vi "Teleop.vi"(10 "Match Info":T1={"Autonomous Elapsed Seconds"=0.0, "TeleOp Elapsed Seconds"=0.0, "Disabled Elapsed Seconds"=0.0, "Visited Autonomous"=FALSE, "Visited TeleOp"=FALSE, "Visited Disabled"=FALSE, "Autonomous Settings"={"Autonomous Style"=enum."Independent", "VI Refnum"=refnum}}, 11 "Call Context":T2) -> ()   [LabVIEW 2019]
doc: "This VI is called for each TeleOp packet received from the DS where the robot is not disabled. It is often used to read from the joysticks and update I/O or to update setpoints for timed control loops. It should complete and return within 20 milliseconds or it may miss DS packets."
uses:
  <vilib>/Rock Robotics/WPI/DriverStation/WPI_DriverStationDerivedRobotMode.ctl
  <vilib>/Rock Robotics/WPI/DriverStation/WPI_DriverStationMatch Info.ctl
  <vilib>/Rock Robotics/WPI/Utilities/WPI_GetSetVariantRefNum.vi
  <vilib>/Rock Robotics/Network Tables/NT Write String.vi
  <vilib>/Rock Robotics/Network Tables/NT Write Number.vi
  <vilib>/Rock Robotics/Network Tables/NT Write Numeric Array.vi
  <vilib>/Rock Robotics/Network Tables/NT Read Boolean.vi
  Robot Global Data.vi
  <vilib>/Rock Robotics/Network Tables/NT Read Number.vi
  <vilib>/Rock Robotics/Network Tables/NT Write Boolean Array.vi
panel:
  in  "Yellow":cluster{"R":dbl, "G":dbl, "B":dbl}
  in  "Blue":cluster{"R":dbl, "G":dbl, "B":dbl}
  in  "Green":cluster{"R":dbl, "G":dbl, "B":dbl}
  in  "Red":cluster{"R":dbl, "G":dbl, "B":dbl}
  in  "None":cluster{"R":dbl, "G":dbl, "B":dbl}
  in  "None":cluster{"R":dbl, "G":dbl, "B":dbl}
  out "Sample Slider 0":dbl(slide) scale=0.0..5.0
  out "Sample Boolean 1":bool
  out "Sample Boolean 0":bool
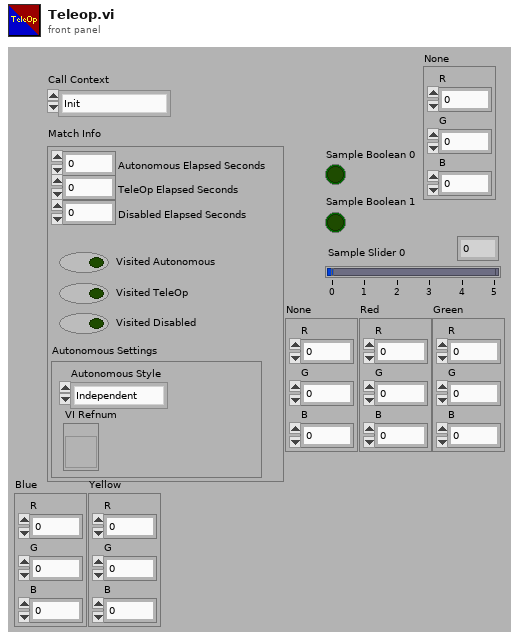
[diagram p1: front panel]
types:
  T1 = typedef "WPI_DriverStationMatch Info.ctl" = cluster{"Autonomous Elapsed Seconds":dbl, "TeleOp Elapsed Seconds":dbl, "Disabled Elapsed Seconds":dbl, "Visited Autonomous":bool, "Visited TeleOp":bool, "Visited Disabled":bool, "Autonomous Settings":cluster{"Autonomous Style":enum16{"Iterative", "Independent"}, "VI Refnum":refnum<vi>}}
  T2 = typedef "WPI_DriverStationDerivedRobotMode.ctl" = enum16{"Init", "Execute", "Stop"}
  T3 = typedef "WPI_RobotDriveDevRef.ctl" = cluster{"DevStatus":errorcluster, "Motors[]":T4[], "Square Inputs":bool, "Max Output":dbl}
  T4 = typedef "WPI_MotorControlDeviceRef.ctl" = cluster{"DeviceStatus":errorcluster, "Type":T5, "PWM":cluster{"PWM Channel":T6, "DeadBand":T7}, "CAN":cluster{"Device Number":u8, "SetOutput VI Ref":variant, "GetOutput VI Ref":variant, "Enable VI Ref":variant, "Disable VI Ref":variant, "Data":variant}, "Invert":bool, "DIO PWM":cluster{"PWM \"Enable\" Channel":T6, "DIOChannel":T8, "PWM Rate":dbl}}
  T5 = typedef "WPI_MotorControlType.ctl" = enum16{"PWM", "CAN", "DIO PWM"}
  T6 = typedef "FPGA_DIOPWMChannel.ctl" = enum8{"PWM 0", "PWM 1", "PWM 2", "PWM 3", "PWM 4", "PWM 5", "PWM 6", "PWM 7", "PWM 8", "PWM 9", "PWM MXP 0", "PWM MXP 1", "PWM MXP 2", "PWM MXP 3", "PWM MXP 4", "PWM MXP 5", "PWM MXP 6", "PWM MXP 7", "PWM MXP 8", "PWM MXP 9", "Invalid"}
  T7 = typedef "WPI_PWMDeadband.ctl" = cluster{"Name":string, "maxPositivePwm":i32, "minPositivePwm":i32, "centerPwm":i32, "maxNegativePwm":i32, "minNegativePwm":i32, "angularRange":u16}
  T8 = typedef "FPGA_DIOChannel.ctl" = enum8{"DIO 0", "DIO 1", "DIO 2", "DIO 3", "DIO 4", "DIO 5", "DIO 6", "DIO 7", "DIO 8", "DIO 9", "DIO MXP 0", "DIO MXP 1", "DIO MXP 2", "DIO MXP 3", "DIO MXP 4", "DIO MXP 5", "DIO MXP 6", "DIO MXP 7", "DIO MXP 8", "DIO MXP 9", "DIO MXP 10", "DIO MXP 11", "DIO MXP 12", "DIO MXP 13", "DIO MXP 14", "DIO MXP 15", "SPI Port CS1", "SPI Port CS2", "SPI Port CS3", "SPI Port MISO", "SPI Port MOSI", "Invalid"}
  T9 = typedef "WPI_JoystickDevRef.ctl" = cluster{"Device":T10}
  T10 = typedef "WPI_JoystickDeviceEnum.ctl" = enum16{"USB 0", "USB 1", "USB 2", "USB 3", "USB 4", "USB 5"}
  T11 = cluster{"JoystickDevRef":T9, "RobotDriveDevRef":T3}
  T12 = typedef "Color Sensor V3 DevRef.ctl" = cluster{"I2CDevRef":T13}
  T13 = typedef "WPI_I2CDevRef.ctl" = cluster{"DevStatus":errorcluster, "Device Address":u8, "Handle":i32, "I2C Bus":T14}
  T14 = typedef "i2c_bus.ctl" = enum16{"I2C On-Board", "I2C MXP", "Invalid"}
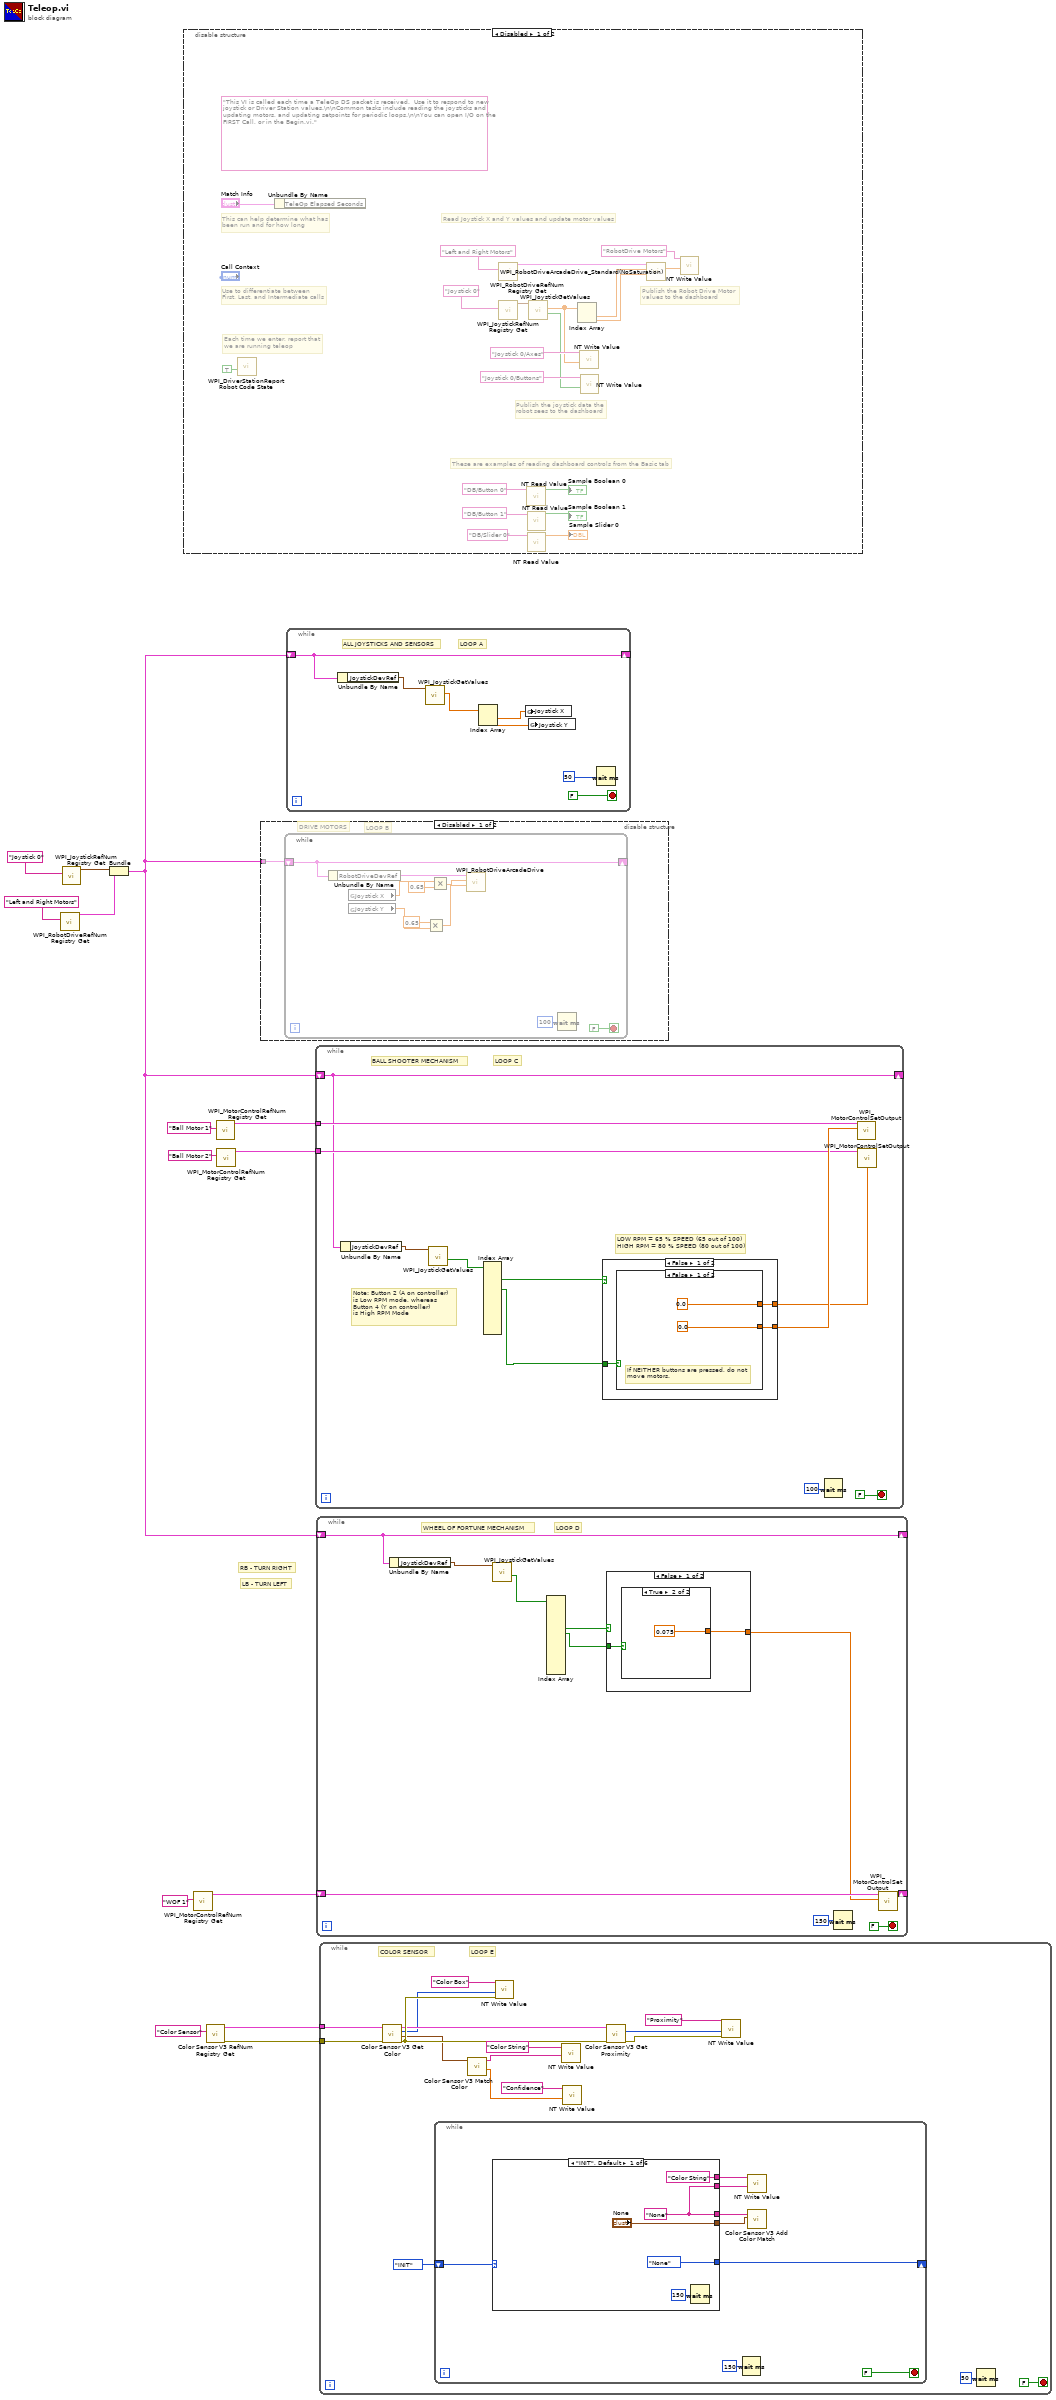
[diagram p0: block diagram]
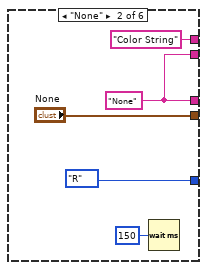
[diagram p4: hidden frame]
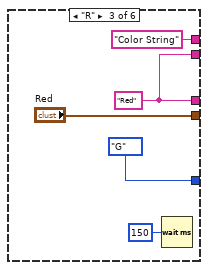
[diagram p5: hidden frame]
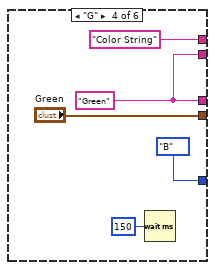
[diagram p6: hidden frame]
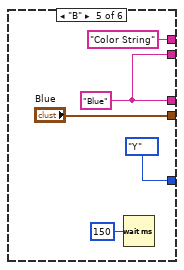
[diagram p7: hidden frame]
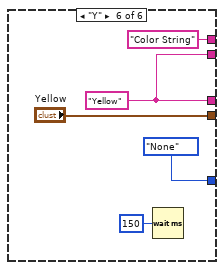
[diagram p8: hidden frame]
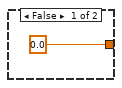
[diagram p9: hidden frame]
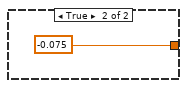
[diagram p10: hidden frame]
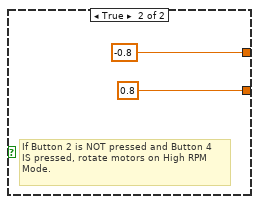
[diagram p11: hidden frame]
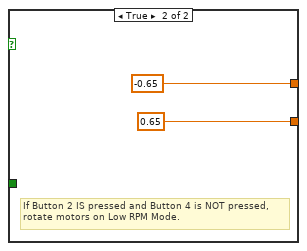
[diagram p12: hidden frame]
diagram:
  # "LB - TURN LEFT"
  # "RB - TURN RIGHT"
  n1 = call <vilib>:"WPI_RobotDriveRefNum Registry Get.vi"("refnum name"="Left and Right Motors") -> ("RobotDriveDevRef"=w11:T3)  [unwired: 1 in, 9 out]
  n2 = call <vilib>:"WPI_JoystickRefNum Registry Get.vi"("refnum name"="Joystick 0") -> ("JoystickDevRef"=w12:T9)  [unwired: 1 in, 9 out]
  n3 = Bundle("JoystickDevRef"=w12, "RobotDriveDevRef"=w11) -> (w1:T11)  [unwired: 1 out]
  n4 = disable-structure shown="Disabled" {
    frame Disabled {
      (unwired) "This VI is called each time a TeleOp DS packet is received.  Use it to respond to new joystick or Driver Station values.\n\nCommon tasks include reading the joysticks and updating motors, and updating setpoints for periodic loops.\n\nYou can open I/O on the FIRST Call, or in the Begin.vi."
      # "These are examples of reading dashboard controls from the Basic tab"
      # "Publish the Robot Drive Motor\nvalues to the dashboard"
      # "Publish the joystick data the\nrobot sees to the dashboard"
      # "Each time we enter, report that\nwe are running teleop"
      # "Use to differentiate between\nFirst, Last, and Intermediate calls"
      # "This can help determine what has\nbeen run and for how long"
      # "Read Joystick X and Y values and update motor values"
      n5 = call <vilib>:"WPI_DriverStationReport Robot Code State.vi"("TeleOp"=TRUE ("Autonomous")) -> ()  [unwired: 10 in, 1 out]
      n6 = Unbundle By Name("Match Info") -> ()  [unwired: 1 out]
      n7 = call <vilib>:"WPI_RobotDriveRefNum Registry Get.vi"("refnum name"="Left and Right Motors") -> ("RobotDriveDevRef"=w32:T3)  [unwired: 1 in, 9 out]
      n8 = call <vilib>:"WPI_JoystickRefNum Registry Get.vi"("refnum name"="Joystick 0") -> ("JoystickDevRef"=w29:T9)  [unwired: 1 in, 9 out]
      n9 = call-poly <vilib>:"NT Read Value.vi"("Name"="DB/Button 0" ("refnum name")) -> ("Boolean"=→"Sample Boolean 0":bool)  [unwired: 9 in, 1 out]
      n10 = call-poly <vilib>:"NT Read Value.vi"("Name"="DB/Button 1" ("refnum name")) -> ("Boolean"=→"Sample Boolean 1":bool)  [unwired: 9 in, 1 out]
      n11 = call-poly <vilib>:"NT Read Value.vi"("Name"="DB/Slider 0" ("refnum name")) -> ("Numeric"=→"Sample Slider 0":dbl)  [unwired: 9 in, 1 out]
      n12 = call <vilib>:"WPI_JoystickGetValues.vi"("JoystickDevRef"=w29) -> ("Buttons"=w23:bool[], "Axes"=w24:dbl[])  [unwired: 6 in, 3 out]
      n13 = Index Array(array=w24) -> (element #1=w31:dbl, element #2=w27:dbl)  [unwired: 2 in]
      n14 = call-poly <vilib>:"NT Write Value.vi"("Numeric Array"=w24, "Name"="Joystick 0/Axes") -> ()  [unwired: 9 in, 1 out]
      n15 = call-poly <vilib>:"NT Write Value.vi"("Boolean Array"=w23, "Name"="Joystick 0/Buttons") -> ()  [unwired: 9 in, 1 out]
      n16 = call <vilib>:"WPI_RobotDriveArcadeDrive_Standard(NoSaturation).vi"("Y axis value"=w27, "X axis value"=w31, "RobotDriveDevRef"=w32) -> ("Motor Values"=w18:dbl[])  [unwired: 1 in, 7 out]
      n17 = call-poly <vilib>:"NT Write Value.vi"("Numeric Array"=w18, "Name"="RobotDrive Motors") -> ()  [unwired: 9 in, 1 out]
    }
    frame Enabled {
    }
  }
  n18 = call <vilib>:"WPI_MotorControlRefNum Registry Get.vi"("refnum name"="WOF 1") -> ("MotorControlDevRef"=w5:T4)  [unwired: 9 in, 1 out]
  n19 = call <vilib>:"Color Sensor V3 RefNum Registry Get.vi"("refnum name"="Color Sensor") -> ("error out"=w2:errorcluster, "ColorSensorDevRef"=w4:T12)  [unwired: 9 in]
  n20 = call <vilib>:"WPI_MotorControlRefNum Registry Get.vi"("refnum name"="Ball Motor 1") -> ("MotorControlDevRef"=w8:T4)  [unwired: 9 in, 1 out]
  n21 = call <vilib>:"WPI_MotorControlRefNum Registry Get.vi"("refnum name"="Ball Motor 2") -> ("MotorControlDevRef"=w7:T4)  [unwired: 9 in, 1 out]
  n22 = disable-structure shown="Disabled" {
    disable-tunnel: w1 -> [w35 _]
    frame Disabled {
      # "LOOP B"
      # "DRIVE MOTORS"
      n23 = while {
        shift-right: [w43] -> _
        shift-left: w35 -> [w43]
        stop <- FALSE stop-if-true
        n24 = Unbundle By Name(w43) -> ("RobotDriveDevRef"=w42:T3)
        n25 = global read "Robot Global Data.vi" "Joystick X"() -> (w40:dbl)
        n26 = global read "Robot Global Data.vi" "Joystick Y"() -> (w41:dbl)
        n27 = Multiply(x=0.65, y=w41) -> (x*y=w37:dbl)
        n28 = Multiply(x=w40, y=0.65) -> (x*y=w36:dbl)
        n29 = call-poly <vilib>:"WPI_RobotDriveArcadeDrive.vi"("Y axis value"=w37, "X axis value"=w36, "RobotDriveDevRef"=w42) -> ()  [unwired: 6 in, 3 out]
        n30 = Wait (ms)(milliseconds to wait=u32 100) -> ()  [unwired: 1 out]
      }
    }
    frame Enabled {
    }
  }
  n31 = while {
    shift-right: [w51] -> _
    shift-left: w1 -> [w51]
    stop <- FALSE stop-if-true
    # "LOOP A"
    # "ALL JOYSTICKS AND SENSORS"
    n32 = Unbundle By Name(w51) -> ("JoystickDevRef"=w50:T9)
    n33 = call <vilib>:"WPI_JoystickGetValues.vi"("JoystickDevRef"=w50) -> ("Axes"=w49:dbl[])  [unwired: 6 in, 4 out]
    n34 = Index Array(array=w49) -> (element #1=w47:dbl, element #2=w48:dbl)  [unwired: 2 in]
    n35 = global write "Robot Global Data.vi" "Joystick X"(w47) -> ()
    n36 = global write "Robot Global Data.vi" "Joystick Y"(w48) -> ()
    n37 = Wait (ms)(milliseconds to wait=u32 50) -> ()  [unwired: 1 out]
  }
  n38 = while {
    shift-right: [w57] -> _
    shift-left: w1 -> [w57]
    tunnel: w8 -> [w61]
    tunnel: w7 -> [w58]
    stop <- FALSE stop-if-true
    # "LOW RPM = 65 % SPEED (65 out of 100)\nHIGH RPM = 80 % SPEED (80 out of 100)"
    # "LOOP C"
    # "Note: Button 2 (A on controller) \nis Low RPM mode, whereas \nButton 4 (Y on controller)\nis High RPM Mode"
    # "BALL SHOOTER MECHANISM"
    n39 = Unbundle By Name(w57) -> ("JoystickDevRef"=w56:T9)
    n40 = call <vilib>:"WPI_JoystickGetValues.vi"("JoystickDevRef"=w56) -> ("Buttons"=w55:bool[])  [unwired: 6 in, 4 out]
    n41 = Index Array(array=w55) -> (element #2=w53:bool, element #4=w54:bool)  [unwired: 13 in, 11 out]
    n42 = case shown="False" w53 {
      tunnel: [w66 0.65 ("Output")] -> w60
      tunnel: [w65 -0.65 ("Output")] -> w59
      tunnel: w54 -> [w64 _]
      frame False {
        n43 = case shown="False" w64 {
          tunnel: [0.0 ("Output") 0.8 ("Output")] -> w66
          tunnel: [0.0 ("Output") -0.8 ("Output")] -> w65
          frame False {
            # "If NEITHER buttons are pressed, do not\nmove motors."
          }
          frame True {
            # "If Button 2 is NOT pressed and Button 4\nIS pressed, rotate motors on High RPM\nMode."
          }
        }
      }
      frame True {
        # "If Button 2 IS pressed and Button 4 is NOT pressed,\nrotate motors on Low RPM Mode."
      }
    }
    n44 = Wait (ms)(milliseconds to wait=u32 100) -> ()  [unwired: 1 out]
    n45 = call <vilib>:"WPI_MotorControlSetOutput.vi"("Output"=w60, "MotorControlDevRef"=w61) -> ()  [unwired: 7 in, 3 out]
    n46 = call <vilib>:"WPI_MotorControlSetOutput.vi"("Output"=w59, "MotorControlDevRef"=w58) -> ()  [unwired: 7 in, 3 out]
  }
  n47 = while {
    shift-right: [w81] -> _
    shift-left: w1 -> [w81]
    shift-right: [w77] -> _
    shift-left: w5 -> [w78]
    stop <- FALSE stop-if-true
    # "LOOP D"
    # "WHEEL OF FORTUNE MECHANISM"
    n48 = Unbundle By Name(w81) -> ("JoystickDevRef"=w80:T9)
    n49 = call <vilib>:"WPI_JoystickGetValues.vi"("JoystickDevRef"=w80) -> ("Buttons"=w79:bool[])  [unwired: 6 in, 4 out]
    n50 = Index Array(array=w79) -> (element #5=w75:bool, element #6=w74:bool)  [unwired: 14 in, 12 out]
    n51 = case shown="False" w75 {
      tunnel: [w83 -0.075 ("Output")] -> w76
      tunnel: w74 -> [w84 _]
      frame False {
        n52 = case shown="True" w84 {
          tunnel: [0.0 ("Output") 0.075 ("Output")] -> w83
          frame False {
          }
          frame True {
          }
        }
      }
      frame True {
      }
    }
    n53 = Wait (ms)(milliseconds to wait=u32 150) -> ()  [unwired: 1 out]
    n54 = call <vilib>:"WPI_MotorControlSetOutput.vi"("Output"=w76, "MotorControlDevRef"=w78) -> ("MotorControlDevRef"=w77:T4)  [unwired: 7 in, 2 out]
  }
  n55 = while {
    tunnel: w4 -> [w103]
    tunnel: w2 -> [w102]
    stop <- FALSE stop-if-true
    # "LOOP E"
    # "COLOR SENSOR"
    n56 = call <vilib>:"Color Sensor V3 Get Color.vi"("error in (no error)"=w102, "ColorSensorDevRef"=w103) -> ("error out"=w101:errorcluster, "Normalized Color"=w95:cluster{"R":dbl, "G":dbl, "B":dbl}, "Color"=w98:u32, "ColorSensorDevRef out"=w99:T12)  [unwired: 6 in]
    n57 = while {
      shift-right: [w109] -> _
      shift-left: enum16{"INIT", "None", "R", "G", "B", "Y"}."INIT" -> [w110]
      stop <- FALSE stop-if-true
      n58 = case shown="\"INIT\", Default" w110 {
        tunnel: [enum16{"INIT", "None", "R", "G", "B", "Y"}."None" enum16{"INIT", "None", "R", "G", "B", "Y"}."R" enum16{"INIT", "None", "R", "G", "B", "Y"}."G" enum16{"INIT", "None", "R", "G", "B", "Y"}."B" enum16{"INIT", "None", "R", "G", "B", "Y"}."Y" enum16{"INIT", "None", "R", "G", "B", "Y"}."None"] -> w109
        tunnel: [w115 w120 w125 w132 w136 w141] -> w108
        tunnel: [w115 w120 w125 w132 w136 w141] -> w107
        tunnel: ["Color String" ("Name") "Color String" ("Name") "Color String" ("Name") "Color String" ("Name") "Color String" ("Name") "Color String" ("Name")] -> w106
        tunnel: ["None" "None" "Red" "Green" "Blue" "Yellow"] -> w105
        frame "INIT", Default {
          w115 = "None" ("Name")
          n59 = Wait (ms)(milliseconds to wait=u32 150) -> ()  [unwired: 1 out]
        }
        frame "None" {
          w120 = "None" ("Name")
          n60 = Wait (ms)(milliseconds to wait=u32 150) -> ()  [unwired: 1 out]
        }
        frame "R" {
          w125 = "Red" ("Name")
          n61 = Wait (ms)(milliseconds to wait=u32 150) -> ()  [unwired: 1 out]
        }
        frame "G" {
          w132 = "Green" ("Name")
          n62 = Wait (ms)(milliseconds to wait=u32 150) -> ()  [unwired: 1 out]
        }
        frame "B" {
          w136 = "Blue" ("Name")
          n63 = Wait (ms)(milliseconds to wait=u32 150) -> ()  [unwired: 1 out]
        }
        frame "Y" {
          w141 = "Yellow" ("Name")
          n64 = Wait (ms)(milliseconds to wait=u32 150) -> ()  [unwired: 1 out]
        }
      }
      n65 = Wait (ms)(milliseconds to wait=u32 150) -> ()  [unwired: 1 out]
      n66 = call-poly <vilib>:"NT Write Value.vi"("String"=w107, "Name"=w106) -> ()  [unwired: 9 in, 1 out]
      n67 = call <vilib>:"Color Sensor V3 Add Color Match.vi"("Color"=w105, "Name"=w108) -> ()  [unwired: 10 in]
    }
    n68 = call <vilib>:"Color Sensor V3 Match Color.vi"("Measured Color"=w95) -> ("Confidence"=w94:dbl, "Matched Color Name"=w93:string)  [unwired: 8 in, 1 out]
    n69 = call-poly <vilib>:"NT Write Value.vi"("error in"=w101, "Numeric"=w98, "Name"="Color Box") -> ()  [unwired: 8 in, 1 out]
    n70 = call-poly <vilib>:"NT Write Value.vi"("String"=w93, "Name"="Color String") -> ()  [unwired: 9 in, 1 out]
    n71 = call-poly <vilib>:"NT Write Value.vi"("Numeric"=w94, "Name"="Confidence") -> ()  [unwired: 9 in, 1 out]
    n72 = call <vilib>:"Color Sensor V3 Get Proximity.vi"("error in (no error)"=w101, "ColorSensorDevRef"=w99) -> ("error out"=w96:errorcluster, "Proximity"=w97:u16)  [unwired: 7 in, 1 out]
    n73 = call-poly <vilib>:"NT Write Value.vi"("error in"=w96, "Numeric"=w97, "Name"="Proximity") -> ()  [unwired: 8 in, 1 out]
    n74 = Wait (ms)(milliseconds to wait=u32 50) -> ()  [unwired: 1 out]
  }
